vi "Configure Sweep Coupling Characteristic.vi"(0 "VISA resource name":refnum<visa-resource-name>, 1 "Delay Time (0.003 seconds)":dbl=0.003, 2 "Trigger Source (0: External)":i32(ring) items=["External", "Frame", "RF Burst"], 5 "Enable Gated Sweep (F: Disable)":bool, 7 "Enable Gate View (F: Disable)":bool, 9 "Gated View Time (0.001 seconds)":dbl=0.001, 11 "error in (no error)":errorcluster, 12 "Gate Length (0.5 seconds)":dbl=0.5) -> (4 "VISA resource name out":refnum<visa-resource-name>, 15 "error out":errorcluster)   [LabVIEW 2022 SP3, in "Agilent N934X Series.lvlib"]
doc: "Configure the sweep and coupling settings.\n\nNote:\nThis VI is only applicable for N9321C, N9322C, N9323C, N9324C models."
uses:
  <instrlib>/Agilent N934X Series/Agilent N934X Series.lvlib
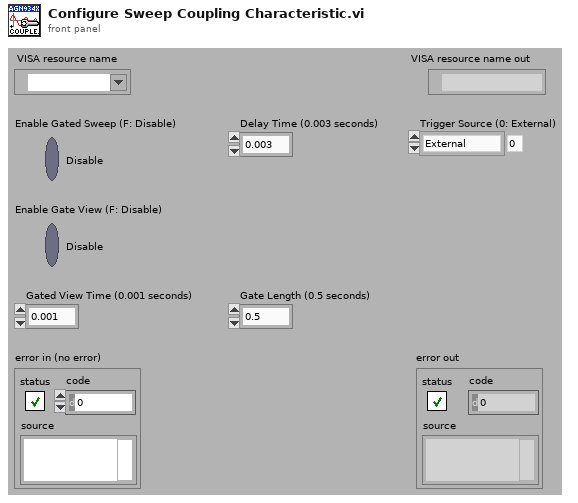
[diagram p1: front panel]
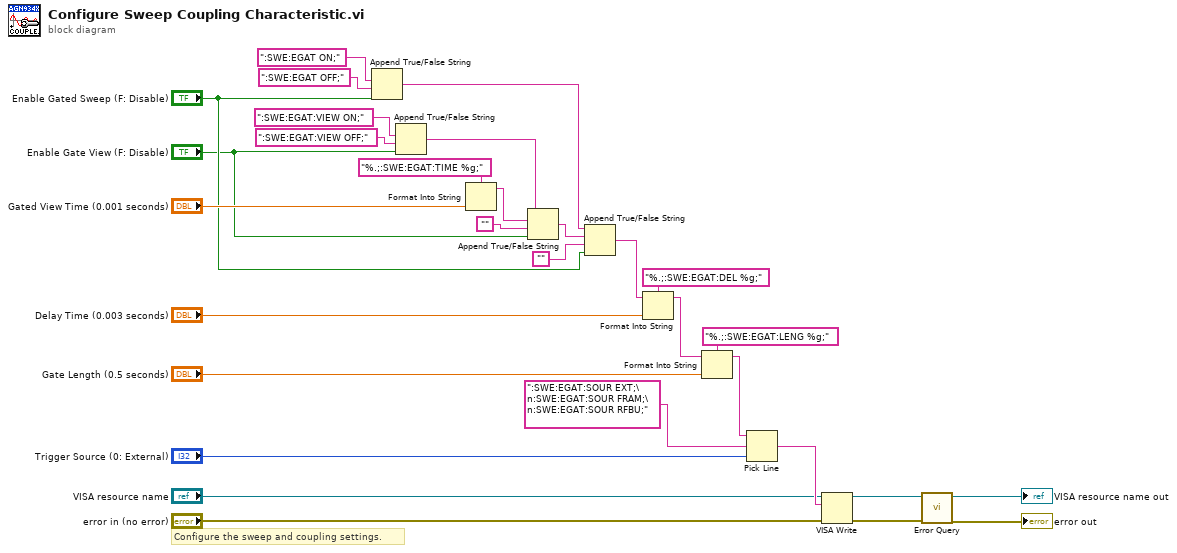
[diagram p0: block diagram]
diagram:
  # "Configure the sweep and coupling settings."
  n1 = Append True/False String(1:"Enable Gated Sweep (F: Disable)", 2:":SWE:EGAT OFF;", 3:":SWE:EGAT ON;") -> (0:w8:string)  [unwired: 1 in]
  n2 = Append True/False String(1:"Enable Gate View (F: Disable)", 2:":SWE:EGAT:VIEW OFF;", 3:":SWE:EGAT:VIEW ON;") -> (0:w4:string)  [unwired: 1 in]
  n3 = Format Into String(format string="%.;:SWE:EGAT:TIME %g;", "Gated View Time (0.001 seconds)") -> (resulting string=w3:string)  [unwired: 2 in, 1 out]
  n4 = Append True/False String(1:"Enable Gate View (F: Disable)", 2:"", 3:w3, 4:w4) -> (0:w1:string)
  n5 = Append True/False String(1:"Enable Gated Sweep (F: Disable)", 2:"", 3:w1, 4:w8) -> (0:w6:string)
  n6 = Format Into String(format string="%.;:SWE:EGAT:DEL %g;", initial string=w6, "Delay Time (0.003 seconds)") -> (resulting string=w22:string)  [unwired: 1 in, 1 out]
  n7 = Format Into String(format string="%.;:SWE:EGAT:LENG %g;", initial string=w22, "Gate Length (0.5 seconds)") -> (resulting string=w17:string)  [unwired: 1 in, 1 out]
  n8 = Pick Line(string ("")=w17, multi-line string=":SWE:EGAT:SOUR EXT;\n:SWE:EGAT:SOUR FRAM;\n:SWE:EGAT:SOUR RFBU;", line index="Trigger Source (0: External)") -> (output string=w16:string)
  n9 = VISA Write(VISA resource name="VISA resource name", write buffer=w16, error in (no error)="error in (no error)") -> (VISA resource name out=w13:refnum<visa-resource-name>, error out=w12:errorcluster)  [unwired: 1 out]
  n10 = call <instrlib>:"Error Query.vi"("error in (no error)"=w12, "VISA resource name"=w13) -> ("error out"=→"error out":errorcluster, "VISA resource name out"=→"VISA resource name out":refnum<visa-resource-name>)  [unwired: 6 in, 2 out]
